vi "Validate From Module Connection Information.vi"(8 "error in (no error)":errorcluster, 10 "Module Connection Information":T1[](array[typedef]), 11 "Routing and Faulting Custom Device Ref in":T3 format="%.0x") -> (0 "error out":errorcluster, 2 "Module Connection Information out":T1[](array[typedef]), 3 "Routing and Faulting Custom Device Ref out":T3 format="%.0x")   [LabVIEW 2017, in "Routing and Faulting Scripting.lvlib"]
uses:
  Routing and Faulting Scripting.lvlib
  Types/Module Connection Information.ctl
  Shared/Routing and Faulting Hardware API/Types/Possible Connections for Endpoint.ctl
  <vilib>/NI Veristand/Custom Device API/Custom Device Item Ref.ctl
  Shared/Routing and Faulting Hardware API/Routing and Faulting Hardware API.lvlib
  <vilib>/NI Veristand/Custom Device API/Custom Device API.lvlib
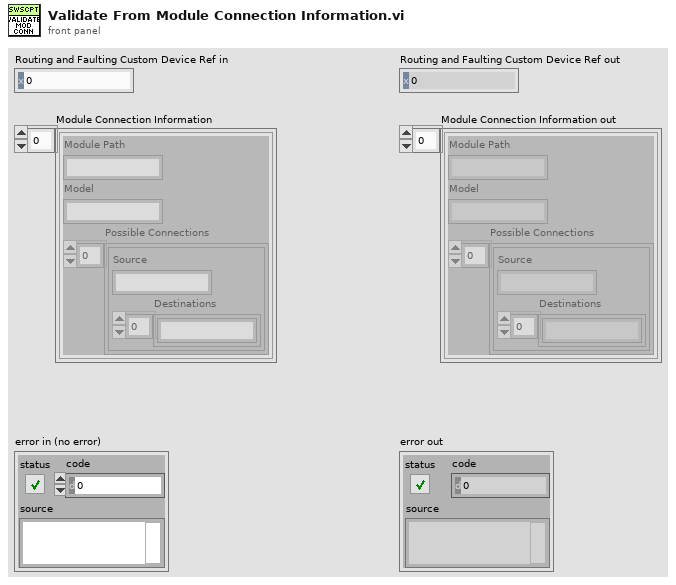
[diagram p1: front panel]
types:
  T1 = typedef "Routing and Faulting Scripting.lvlib/Module Connection Information.ctl" = cluster{"Module Path":string, "Model":string, "Possible Connections":T2[]}
  T2 = typedef "Routing and Faulting Hardware API.lvlib/Possible Connections for Endpoint.ctl" = cluster{"Source":string, "Destinations":string[]}
  T3 = typedef "Custom Device API.lvlib/Custom Device Item Ref.ctl" = u64
  T4 = typedef "Routing and Faulting Scripting.lvlib/Validation Information.ctl" = cluster{"Missing Modules":variant, "Module Connection Map":variant, "Unused Modules":variant}
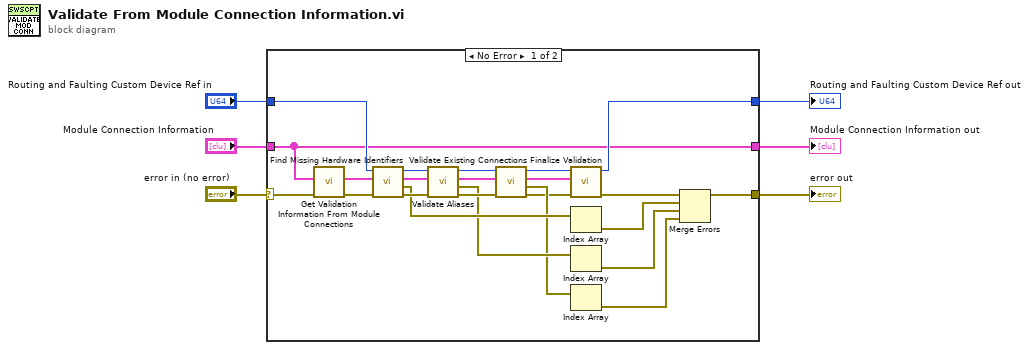
[diagram p0: block diagram]
diagram:
  n1 = case shown="No Error" "error in (no error)" {
    selector: "error in (no error)" -> [w21 w32]
    tunnel: "Module Connection Information" -> [w7 w30]
    tunnel: [w13 w32] -> w5
    tunnel: "Routing and Faulting Custom Device Ref in" -> [w23 w31]
    tunnel: [w8 w31] -> w2
    tunnel: [w7 w30] -> w1
    frame No Error {
      n2 = call "Get Validation Information From Module Connections.vi"("error in (no error)"=w21, "Module Connection Information"=w7) -> ("error out"=w22:errorcluster, "Validation Information"=w20:T4)  [unwired: 8 in]
      n3 = call "Find Missing Hardware Identifiers.vi"("error in (no error)"=w22, "Validation Information in"=w20, "Routing and Faulting Custom Device Ref in"=w23) -> ("error out"=w29:errorcluster, "Identifier Errors"=w19:errorcluster[], "Validation Information out"=w25:T4, "Routing and Faulting Custom Device Ref out"=w28:T3)  [unwired: 5 in]
      n4 = call "Validate Aliases.vi"("error in (no error)"=w29, "Validation Information in"=w25, "Routing and Faulting Custom Device Ref in"=w28) -> ("error out"=w27:errorcluster, "Aliases Errors"=w18:errorcluster[], "Validation Information out"=w24:T4, "Routing and Faulting Custom Device Ref out"=w26:T3)  [unwired: 5 in]
      n5 = call "Validate Existing Connections.vi"("error in (no error)"=w27, "Validation Information in"=w24, "Routing and Faulting Custom Device Ref in"=w26) -> ("error out"=w12:errorcluster, "Connection Errors"=w17:errorcluster[], "Validation Information out"=w9:T4, "Routing and Faulting Custom Device Ref out"=w10:T3)  [unwired: 5 in]
      n6 = call "Finalize Validation.vi"("error in (no error)"=w12, "Validation Information in"=w9, "Routing and Faulting Custom Device Ref in"=w10) -> ("error out"=w11:errorcluster, "Routing and Faulting Custom Device Ref out"=w8:T3)  [unwired: 7 in]
      n7 = Index Array(array=w19) -> (element=w16:errorcluster)  [unwired: 1 in]
      n8 = Index Array(array=w18) -> (element=w15:errorcluster)  [unwired: 1 in]
      n9 = Index Array(array=w17) -> (element=w14:errorcluster)  [unwired: 1 in]
      n10 = Merge Errors(w11, w16, w15, w14) -> (w13:errorcluster)
    }
    frame Error {
    }
  }
  "error out" <- w5
  "Routing and Faulting Custom Device Ref out" <- w2
  "Module Connection Information out" <- w1
